vi "Get IDs or Error.vi"(0 "RegisteredHandler JSON in":refnum<class "RegisteredHandler JSON.lvclass">, 11 "error in (no error)":errorcluster) -> (4 "RegisteredHandler JSON out":refnum<class "RegisteredHandler JSON.lvclass">, 6 "Request ID":u64, 8 "Registration ID":u64, 10 "ErrorOrSuccess":refnum<class "ErrorOrSuccess.lvclass">, 15 "error out":errorcluster)   [LabVIEW 2020, in "wamplv.lvlib" / "RegisteredHandler JSON.lvclass"]
uses:
  RegisteredHandler JSON.lvclass
  RegisteredHandler JSON.lvclass/RegisteredHandler JSON.ctl
  SerialisedMessages/JSONMessage/WampMessage JSON.lvclass
  Error/ErrorHandler JSON/ErrorHandler JSON.lvclass
  <vilib>/Utility/error.llb/Error Cluster From Error Code.vi
  <vilib>/ErrorRing/Error Ring.xnode
  Message loop classes/ErrorOrSuccess JSON/ErrorOrSuccess JSON.lvclass
  C:/local/wamplv/Private/Message loop classes/ErrorOrSuccess/ErrorOrSuccess.lvclass
  C:/local/wamplv/Private/Message loop classes/ErrorOrSuccess JSON/ErrorOrSuccess JSON.lvclass
  Message loop classes/ErrorOrSuccess/ErrorOrSuccess.lvclass
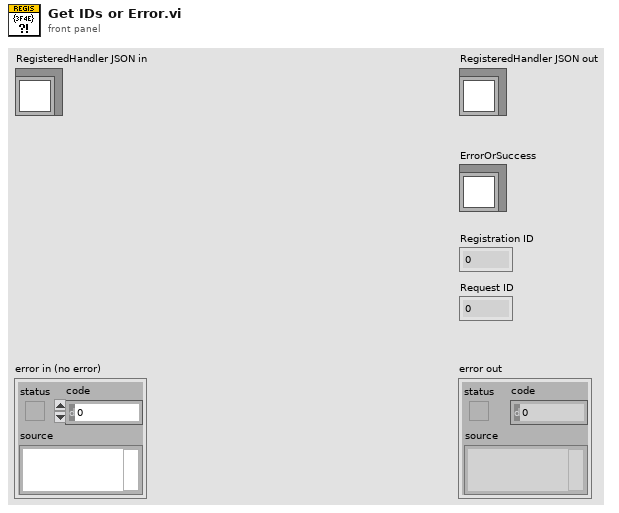
[diagram p1: front panel]
types:
  T1 = typedef "wamplv.lvlib/WAMP Message Codes.ctl" = enum8{"HELLO", "WELCOME", "CHALLENGE", "AUTHENTICATE", "ABORT", "GOODBYE", "ERROR", "PUBLISH", "PUBLISHED", "SUBSCRIBE", "SUBSCRIBED", "UNSUBSCRIBE", "UNSUBSCRIBED", "EVENT", "CALL", "RESULT", "REGISTER", "REGISTERED", "UNREGISTER", "UNREGISTERED", "INVOCATION", "YIELD"}
  T2 = typedef "wamplv.lvlib/Error (JSON).ctl" = cluster{"Request ID":u64, "Message type that caused error":T1, "Error/Abort details (JSON)":T3}
  T3 = typedef "wamplv.lvlib/Error or abort detail (JSON).ctl" = cluster{"Error URI":string, "Error Arguments":string, "Error ArgumentKw":string, "Error Details":string, "Associated LabVIEW Error":errorcluster}
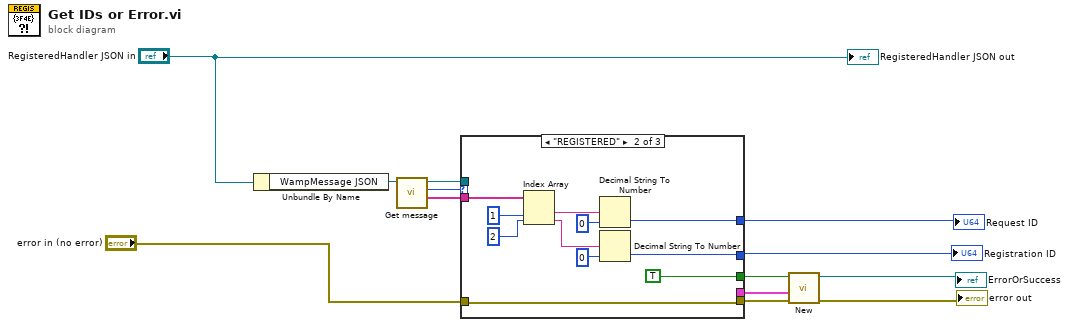
[diagram p0: block diagram]
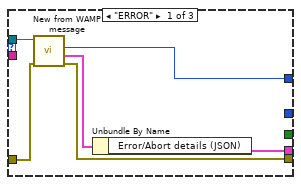
[diagram p2: hidden frame]
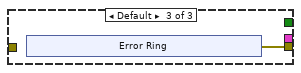
[diagram p3: hidden frame]
diagram:
  n1 = Unbundle By Name("RegisteredHandler JSON in") -> ("WampMessage JSON"=w13:refnum<class "WampMessage JSON.lvclass">)
  n2 = call "Get message.vi"("JSONMessage in"=w13) -> ("<JSON>Elements"=w10:string[], "Message Type"=w12:T1, "JSONMessage out"=w11:refnum<class "WampMessage JSON.lvclass">)  [unwired: 8 in]
  n3 = case shown="\"REGISTERED\"" w12 {
    tunnel: w11 -> [w19 _ _]
    tunnel: w10 -> [_ w27 _]
    tunnel: [w18 w26 _] -> w2
    tunnel: [w16 _ _] -> w9
    tunnel: [_ TRUE _] -> w8
    tunnel: "error in (no error)" -> [w15 w24 _]
    tunnel: [w14 w24 w31] -> w7
    tunnel: [_ w20 _] -> w1
    frame "ERROR" {
      n4 = call "New from WAMP message.vi"("error in (no error)"=w15, "wamplv.lvlib:JSONMessage.lvclass"=w19) -> ("error out"=w14:errorcluster, "Error data (JSON)"=w17:T2, "Request ID"=w18:u64)  [unwired: 6 in, 1 out]
      n5 = Unbundle By Name(w17) -> ("Error/Abort details (JSON)"=w16:T3)
    }
    frame "REGISTERED" {
      n6 = Index Array(array=w27, index #1=1 ("index"), index #2=2 ("index")) -> (element #1=w29:string, element #2=w21:string)
      n7 = Decimal String To Number(string=w29, default (0L)=u64 0) -> (number=w26:u64)  [unwired: 1 in, 1 out]
      n8 = Decimal String To Number(string=w21, default (0L)=u64 0) -> (number=w20:u64)  [unwired: 1 in, 1 out]
    }
    frame Default {
      n9 = xnode "Error Ring"() -> ("error out"=w31:errorcluster)
    }
  }
  "Request ID" <- w2
  "Registration ID" <- w1
  n10 = call "New.vi"("error in (no error)"=w7, "Error/Abort details (JSON)"=w9, "Success?"=w8) -> ("error out"=→"error out":errorcluster, "ErrorOrSuccess JSON out"=→"ErrorOrSuccess":refnum<class "ErrorOrSuccess JSON.lvclass">)  [unwired: 7 in]
  "RegisteredHandler JSON out" <- "RegisteredHandler JSON in"
